vi "interfaz.vi"() -> ()   [LabVIEW 2020]
uses:
  posi inicial- proceso 2.vi
  posi inicial-proceso 3.vi
  posi inicial-proceso 6.vi
  posi incial-proceso 4.vi
  posi incial-proceso 5.vi
  posi incial-proceso 1.vi
panel:
  out "Temperatura del tanque":dbl(slide) scale=0.0..150.0
  out "Agua":bool
  out "nivel de tanque- fermentación 2":dbl(slide) scale=0.0..100.0
  out "tuberia 21":bool
  out "tuberia 20":bool
  out "tuberia 14":bool
  out "tuberia 13":bool
  out "Llama":bool
  out "nivel del tanque -cocción":dbl(slide) scale=0.0..100.0
  out "tuberia  11":bool
  out "tuberia 12":bool
  out "tuberia 10":bool
  out "tuberia 9":bool
  out "tuberia 6":bool
  out "Mezcladora":bool
  out "Nivel-Filtrado":dbl(slide) scale=0.0..100.0
  out "tuberia 5":bool
  out "tuberia 7":bool
  out "tuberia 8":bool
  out "Piñon2":bool
  out "piñon1":bool
  out "tuberia 3":bool
  out "tuberia 2":bool
  out "banda":bool
  out "tuberia1":bool
  out "tuberia 25":bool
  out "tuberia 26":bool
  out "tuberia 24":bool
  out "tuberia 23":bool
  out "ventilador de enfriamiento":bool
  out "tuberia 16":bool
  out "tuberia 15":bool
  out "tuberia 17":bool
  out "tuberia 19":bool
  out "tuberia 18":bool
  out "tuberia 4":bool
  out "tuberia 22":bool
  out "Cebada":bool
  # "Enfriado"
  # "Ingreso de cebada"
  # "Filtrado"
  # "Cocción"
  # "Malteado"
  # "Molienda"
  # "Fermentación"
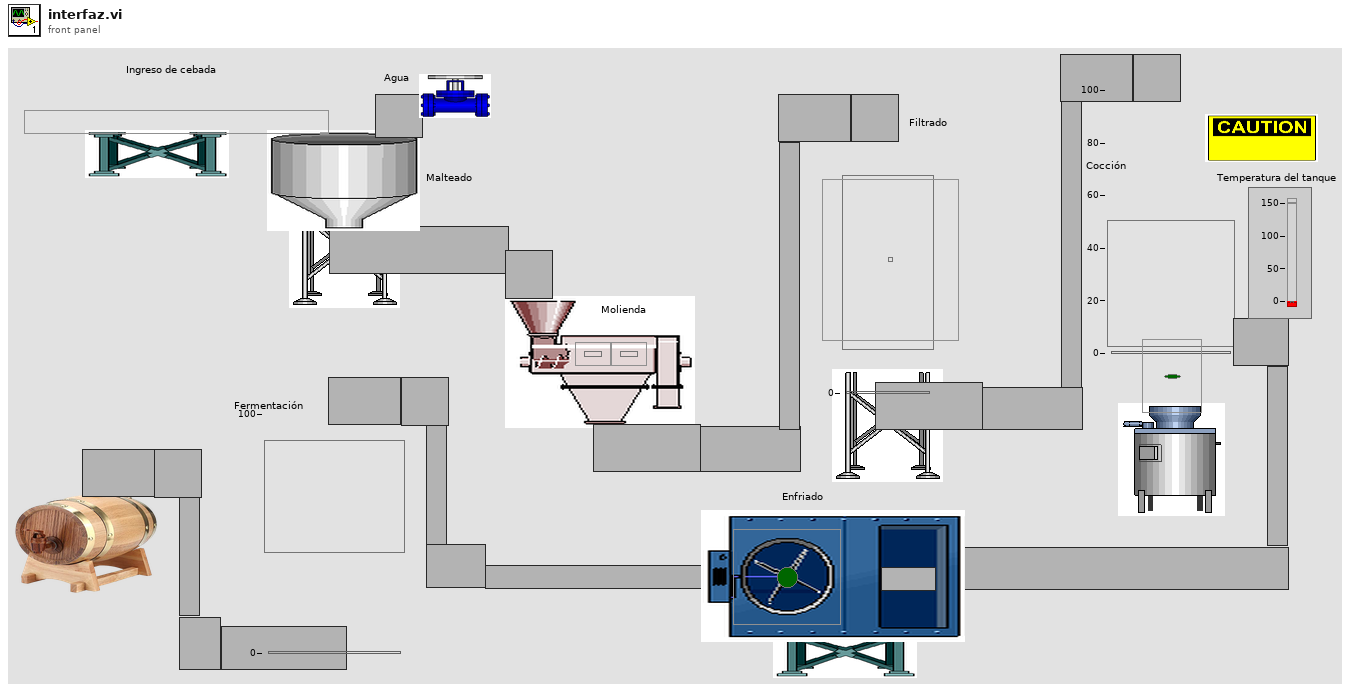
[diagram p1: front panel]
types:
  T1 = cluster{"Posicion  x-cebada":dbl, "banda":bool, "agua":bool, "Posicion y -cebada ":dbl, " visibilida-cebada":bool}
  T2 = cluster{"tuberia 13":bool, "tuberia 14":bool, "tuberia 15":bool, "tuberia 16":bool, "tuberia 17":bool, "tuberia 18":bool, "tuberia 19":bool, "tuberia  20":bool, " ventilador -enfriamiento":bool, "tuberia 21":bool}
  T3 = cluster{"tuberia 8":bool, "tuberia 9":bool, "tuberia 10":bool, "tuberia 11":bool, "tuberia 12":bool, "nivel de cocción":dbl, "Temperatura del tanque":dbl, "llama":bool}
  T4 = cluster{"tuberia 22":bool, "nivel de tanque -fermentación":dbl, "tuberia 23":bool, "tuberia 24":bool, "tuberia 25":bool, "tuberia 26":bool}
  T5 = cluster{"tuberia 3":bool, " tuberia 4":bool, "tuberia 7":bool, "tuberia 5":bool, " tuberia 6":bool, "mezlcadora ":bool, "nivel-filtrado":dbl}
  T6 = cluster{"tuberia 1":bool, "tuberia 2":bool, "piñon 1":bool, "piñon 2":bool}
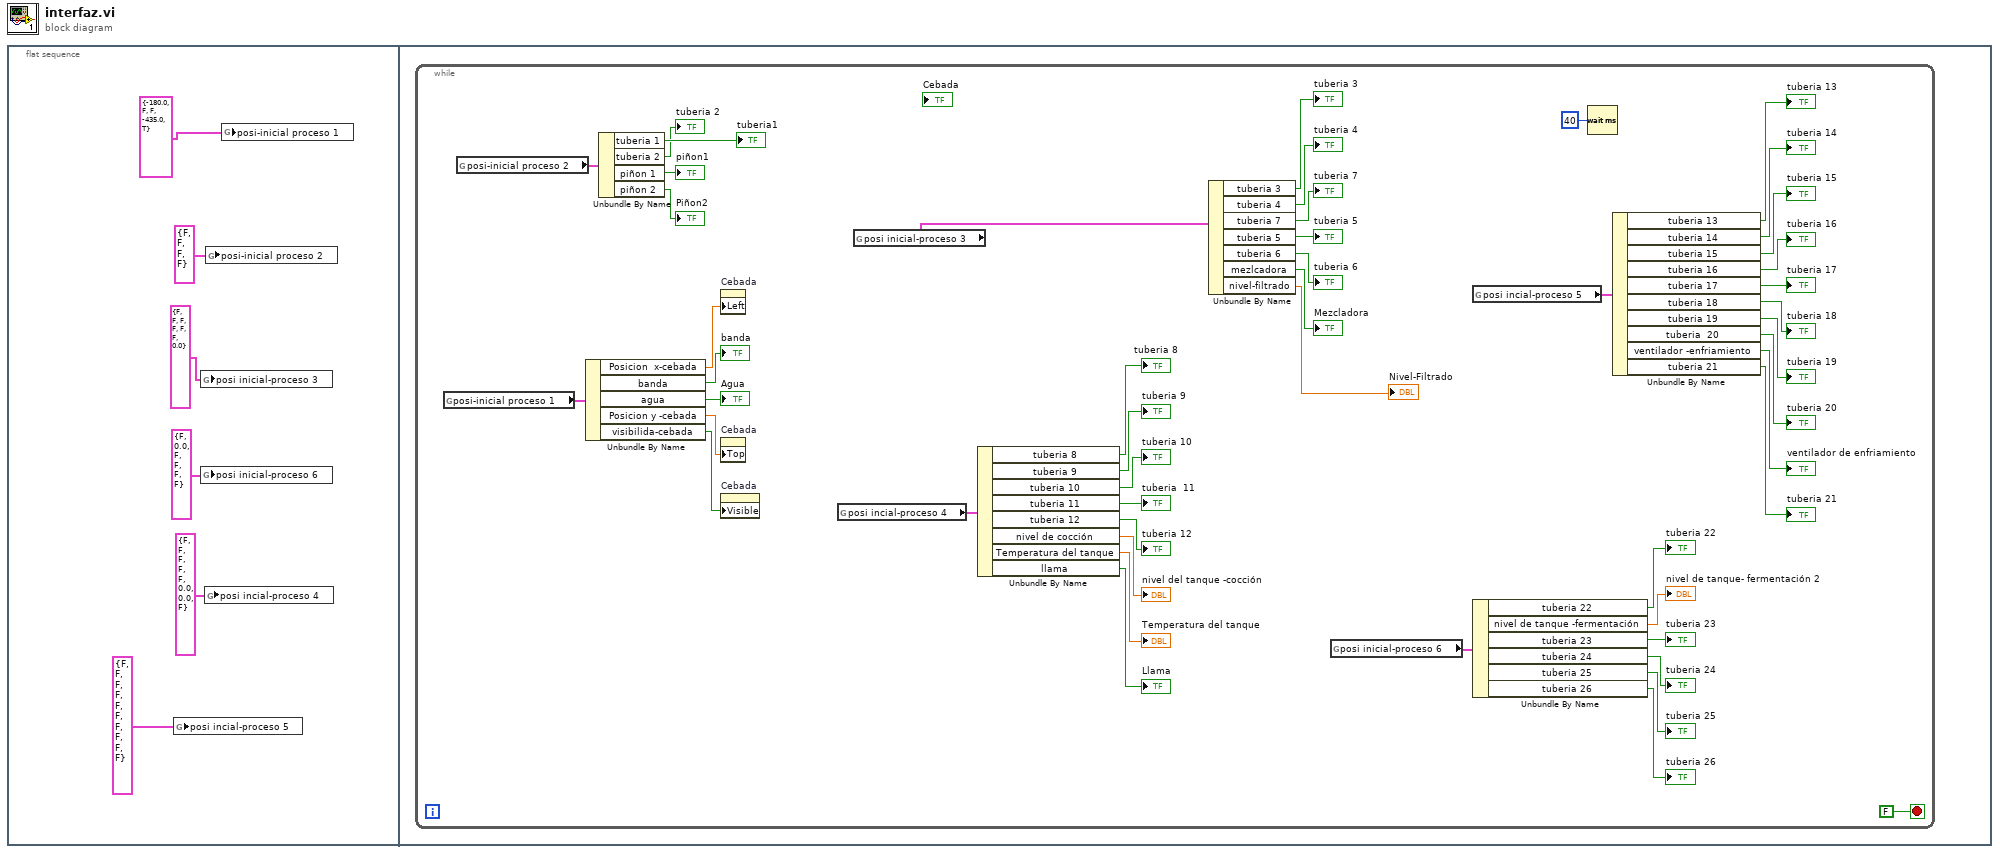
[diagram p0: block diagram]
diagram:
  n1 = flat-sequence {
    frame #0 {
      n2 = global write "posi incial-proceso 5.vi" "posi incial-proceso 5"(T2 {"tuberia 13"=FALSE, "tuberia 14"=FALSE, "tuberia 15"=FALSE, "tuberia 16"=FALSE, "tuberia 17"=FALSE, "tuberia 18"=FALSE, "tuberia 19"=FALSE, "tuberia  20"=FALSE, " ventilador -enfriamiento"=FALSE, "tuberia 21"=FALSE} ("posi incial-proceso 5")) -> ()
      n3 = global write "posi inicial-proceso 3.vi" "posi inicial-proceso 3"(T5 {"tuberia 3"=FALSE, " tuberia 4"=FALSE, "tuberia 7"=FALSE, "tuberia 5"=FALSE, " tuberia 6"=FALSE, "mezlcadora "=FALSE, "nivel-filtrado"=0.0} ("posi inicial-proceso 3")) -> ()
      n4 = global write "posi inicial-proceso 6.vi" "posi inicial-proceso 6"(T4 {"tuberia 22"=FALSE, "nivel de tanque -fermentación"=0.0, "tuberia 23"=FALSE, "tuberia 24"=FALSE, "tuberia 25"=FALSE, "tuberia 26"=FALSE} ("posi inicial-proceso 6")) -> ()
      n5 = global write "posi incial-proceso 4.vi" "posi incial-proceso 4"(T3 {"tuberia 8"=FALSE, "tuberia 9"=FALSE, "tuberia 10"=FALSE, "tuberia 11"=FALSE, "tuberia 12"=FALSE, "nivel de cocción"=0.0, "Temperatura del tanque"=0.0, "llama"=FALSE} ("posi incial-proceso 4")) -> ()
      n6 = global write "posi inicial- proceso 2.vi" "posi-inicial proceso 2"(T6 {"tuberia 1"=FALSE, "tuberia 2"=FALSE, "piñon 1"=FALSE, "piñon 2"=FALSE} ("posi-inicial proceso 2")) -> ()
      n7 = global write "posi incial-proceso 1.vi" "posi-inicial proceso 1"(T1 {"Posicion  x-cebada"=-180.0, "banda"=FALSE, "agua"=FALSE, "Posicion y -cebada "=-435.0, " visibilida-cebada"=TRUE} ("posi-inicial proceso 1")) -> ()
    }
    frame #1 {
      n8 = while {
        stop <- FALSE stop-if-true
        n9 = global read "posi incial-proceso 1.vi" "posi-inicial proceso 1"() -> (w12:T1)
        n10 = global read "posi inicial- proceso 2.vi" "posi-inicial proceso 2"() -> (w54:T6)
        n11 = Unbundle By Name(w12) -> ("Posicion  x-cebada"=w11:dbl, "banda"=→"banda":bool, "agua"=→"Agua":bool, "Posicion y -cebada"=w8:dbl, "visibilida-cebada"=w7:bool)
        n12 = Unbundle By Name(w54) -> ("tuberia 1"=→"tuberia1":bool, "tuberia 2"=→"tuberia 2":bool, "piñon 1"=→"piñon1":bool, "piñon 2"=→"Piñon2":bool)
        n13 = property on="Cebada" class="Bool (strict)"("Left"=w11) -> ()  [unwired: 2 in, 2 out]
        n14 = property on="Cebada" class="Bool (strict)"("Top"=w8) -> ()  [unwired: 2 in, 2 out]
        n15 = property on="Cebada" class="Bool (strict)"("Visible"=w7) -> ()  [unwired: 2 in, 2 out]
        n16 = global read "posi incial-proceso 4.vi" "posi incial-proceso 4"() -> (w41:T3)
        n17 = global read "posi inicial-proceso 3.vi" "posi inicial-proceso 3"() -> (w49:T5)
        n18 = Unbundle By Name(w41) -> ("tuberia 8"=→"tuberia 8":bool, "tuberia 9"=→"tuberia 9":bool, "tuberia 10"=→"tuberia 10":bool, "tuberia 11"=→"tuberia  11":bool, "tuberia 12"=→"tuberia 12":bool, "nivel de cocción"=→"nivel del tanque -cocción":dbl, "Temperatura del tanque"=→"Temperatura del tanque":dbl, "llama"=→"Llama":bool)
        n19 = Unbundle By Name(w49) -> ("tuberia 3"=→"tuberia 3":bool, "tuberia 4"=→"tuberia 4":bool, "tuberia 7"=→"tuberia 7":bool, "tuberia 5"=→"tuberia 5":bool, "tuberia 6"=→"tuberia 6":bool, "mezlcadora"=→"Mezcladora":bool, "nivel-filtrado"=→"Nivel-Filtrado":dbl)
        n20 = global read "posi inicial-proceso 6.vi" "posi inicial-proceso 6"() -> (w21:T4)
        n21 = global read "posi incial-proceso 5.vi" "posi incial-proceso 5"() -> (w32:T2)
        n22 = Unbundle By Name(w21) -> ("tuberia 22"=→"tuberia 22":bool, "nivel de tanque -fermentación"=→"nivel de tanque- fermentación 2":dbl, "tuberia 23"=→"tuberia 23":bool, "tuberia 24"=→"tuberia 24":bool, "tuberia 25"=→"tuberia 25":bool, "tuberia 26"=→"tuberia 26":bool)
        n23 = Wait (ms)(milliseconds to wait=u32 40) -> ()  [unwired: 1 out]
        n24 = Unbundle By Name(w32) -> ("tuberia 13"=→"tuberia 13":bool, "tuberia 14"=→"tuberia 14":bool, "tuberia 15"=→"tuberia 15":bool, "tuberia 16"=→"tuberia 16":bool, "tuberia 17"=→"tuberia 17":bool, "tuberia 18"=→"tuberia 18":bool, "tuberia 19"=→"tuberia 19":bool, "tuberia  20"=→"tuberia 20":bool, "ventilador -enfriamiento"=→"ventilador de enfriamiento":bool, "tuberia 21"=→"tuberia 21":bool)
      }
    }
  }
